vi "is_code_in_range.vi"(4 "code (w/out ECO)":i32) -> (1 "code in allowed range?":bool)   [LabVIEW 2015]
panel:
  # "Some of the error codes are not allowed to be passed to the error handling functions since they are thown by the error handling functions themself"
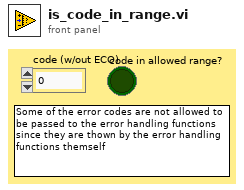
[diagram p1: front panel]
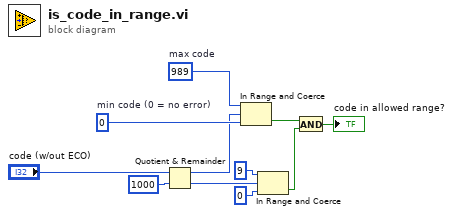
[diagram p0: block diagram]
diagram:
  w11 = 989  # max code
  w10 = 0  # min code (0 = no error)
  n1 = Quotient & Remainder(x="code (w/out ECO)", y=1000) -> (x-y*floor(x/y)=w7:i32, floor(x/y)=w6:i32)
  n2 = In Range and Coerce(upper limit=w11, x=w7, lower limit=w10) -> (In Range?=w4:bool)  [unwired: 1 out]
  n3 = In Range and Coerce(upper limit=9, x=w6, lower limit=0) -> (In Range?=w5:bool)  [unwired: 1 out]
  n4 = And(x=w4, y=w5) -> (x .and. y?=→"code in allowed range?":bool)
